vi "Test_URI_Class_SetPath.vi"(8 "error in (no error)":errorcluster) -> (0 "error out":errorcluster)   [LabVIEW 2013]
uses:
  source/uri/URI.lvclass/URI.ctl
  source/components/path/URI-Component.Path.lvclass/URI-Component.Path.ctl
  source/components/path/Get Segments.vi
  <vilib>/addons/_JKI Toolkits/Caraya/classes/Assert/Assert Equal Value_Variant.vi
  <vilib>/addons/_JKI Toolkits/Caraya/classes/Assert/Assert Error.vi
  source/components/path/Get base-path.vi
  source/components/path/Get path (absolute).vi
  source/components/path/Get path (relative-base).vi
  <vilib>/addons/_JKI Toolkits/Caraya/classes/Test/Test.lvclass
  <vilib>/addons/_JKI Toolkits/Caraya/classes/Assert/Assert.lvclass
  source/uri/URI.lvclass
panel:
  out "Segments":string[](array[string])
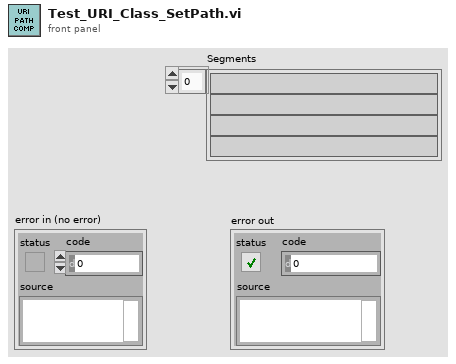
[diagram p1: front panel]
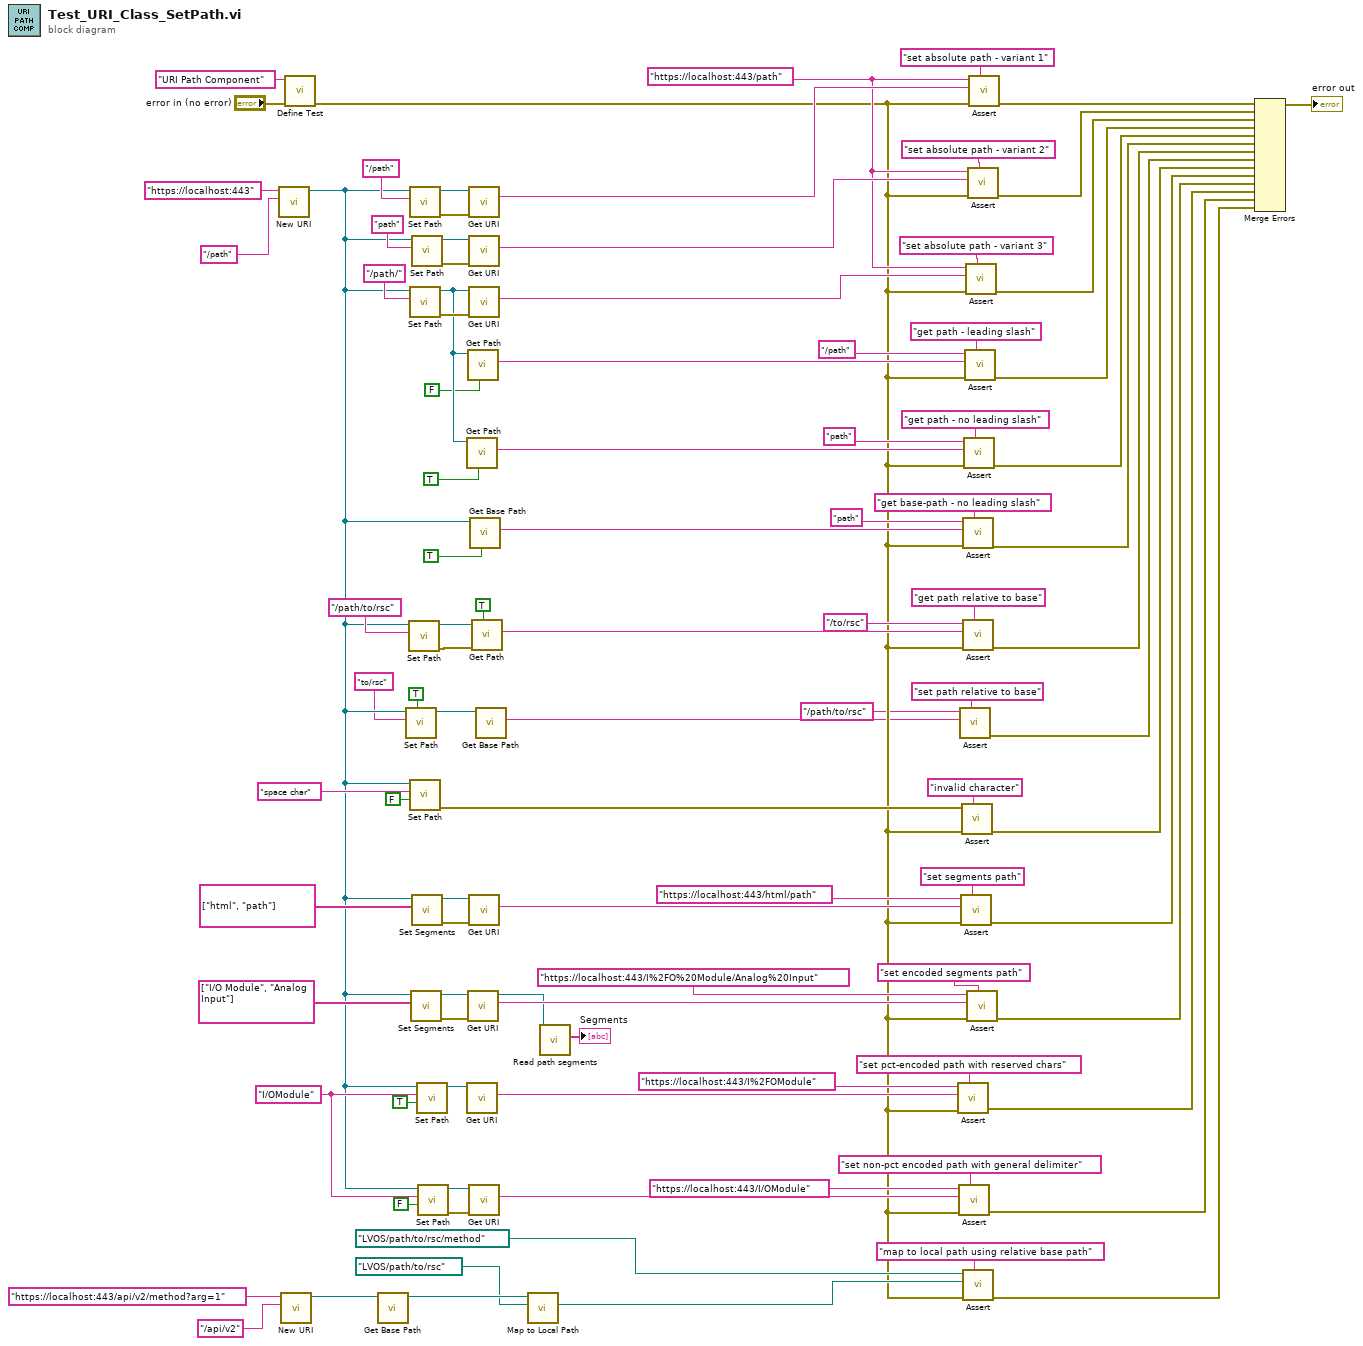
[diagram p0: block diagram]
diagram:
  w75 = "I/OModule" ("URI")
  w90 = "https://localhost:443/path" ("URI")
  n1 = call "New URI.vi"("base-path"="/path" ("URI"), "URI"="https://localhost:443") -> ("URI"=w6:refnum<class "URI.lvclass">)  [unwired: 8 in, 1 out]
  n2 = call "New URI.vi"("base-path"="/api/v2" ("URI"), "URI"="https://localhost:443/api/v2/method?arg=1") -> ("URI"=w22:refnum<class "URI.lvclass">)  [unwired: 8 in, 1 out]
  n3 = call <vilib>:"Define Test.vi"("error in (no error)"="error in (no error)", "Label (VI Title)"="URI Path Component") -> ("error out"=w11:errorcluster)  [unwired: 8 in, 1 out]
  n4 = call "Get Base Path.vi"("URI in"=w22) -> ("URI out"=w24:refnum<class "URI.lvclass">)  [unwired: 8 in, 2 out]
  n5 = call "Set Path.vi"("Use base-path?"=TRUE, "path"="to/rsc" ("URI"), "URI in"=w6) -> ("URI out"=w4:refnum<class "URI.lvclass">)  [unwired: 7 in, 1 out]
  n6 = call "Set Path.vi"("path"="/path/to/rsc" ("URI"), "URI in"=w6) -> ("error out"=w14:errorcluster, "URI out"=w16:refnum<class "URI.lvclass">)  [unwired: 8 in]
  n7 = call "Set Path.vi"("path"="/path" ("URI"), "URI in"=w6) -> ("error out"=w64:errorcluster, "URI out"=w63:refnum<class "URI.lvclass">)  [unwired: 8 in]
  n8 = call "Set Path.vi"("path"="/path/" ("URI"), "URI in"=w6) -> ("error out"=w59:errorcluster, "URI out"=w44:refnum<class "URI.lvclass">)  [unwired: 8 in]
  n9 = call "Set Path.vi"("Encode?"=FALSE, "path"="space char" ("URI"), "URI in"=w6) -> ("error out"=w73:errorcluster)  [unwired: 7 in, 1 out]
  n10 = call "Set Segments.vi"("Segments"=string[] ["I/O Module", "Analog Input"], "URI in"=w6) -> ("error out"=w54:errorcluster, "URI out"=w53:refnum<class "URI.lvclass">)  [unwired: 8 in]
  n11 = call "Set Path.vi"("path"="path" ("URI"), "URI in"=w6) -> ("error out"=w62:errorcluster, "URI out"=w61:refnum<class "URI.lvclass">)  [unwired: 8 in]
  n12 = call "Set Segments.vi"("Segments"=string[] ["html", "path"], "URI in"=w6) -> ("error out"=w55:errorcluster, "URI out"=w56:refnum<class "URI.lvclass">)  [unwired: 8 in]
  n13 = call "Set Path.vi"("Encode?"=TRUE, "path"=w75, "URI in"=w6) -> ("URI out"=w77:refnum<class "URI.lvclass">)  [unwired: 7 in, 1 out]
  n14 = call "Set Path.vi"("Encode?"=FALSE, "path"=w75, "URI in"=w6) -> ("error out"=w71:errorcluster, "URI out"=w70:refnum<class "URI.lvclass">)  [unwired: 7 in]
  n15 = call "Get Path.vi"("Strip lead \"/\" (F)"=TRUE ("Strip lead \"/\" (F)"), "URI in"=w44) -> ("path"=w35:string)  [unwired: 7 in, 2 out]
  n16 = call "Get URI.vi"("URI in"=w77) -> ("URI String"=w80:string)  [unwired: 8 in, 2 out]
  n17 = call "Get Path.vi"("Strip lead \"/\" (F)"=FALSE ("Strip lead \"/\" (F)"), "URI in"=w44) -> ("path"=w40:string)  [unwired: 7 in, 2 out]
  n18 = call "Get URI.vi"("error in (no error)"=w54, "URI in"=w53) -> ("URI String"=w47:string, "URI"=w46:refnum<class "URI.lvclass">)  [unwired: 7 in, 1 out]
  n19 = call "Get URI.vi"("error in (no error)"=w64, "URI in"=w63) -> ("URI String"=w94:string)  [unwired: 7 in, 2 out]
  n20 = call "Get URI.vi"("error in (no error)"=w62, "URI in"=w61) -> ("URI String"=w91:string)  [unwired: 7 in, 2 out]
  n21 = call "Get URI.vi"("error in (no error)"=w59, "URI in"=w44) -> ("URI String"=w89:string)  [unwired: 7 in, 2 out]
  n22 = call "Get URI.vi"("error in (no error)"=w55, "URI in"=w56) -> ("URI String"=w83:string)  [unwired: 7 in, 2 out]
  n23 = call "Get URI.vi"("error in (no error)"=w71, "URI in"=w70) -> ("URI String"=w66:string)  [unwired: 7 in, 2 out]
  n24 = call "Get Base Path.vi"("Strip lead \"/\" (F)"=TRUE ("Strip lead \"/\" (F)"), "URI in"=w6) -> ("base-path"=w28:string)  [unwired: 7 in, 2 out]
  n25 = call "Get Path.vi"("Use base-path?"=TRUE, "error in (no error)"=w14, "URI in"=w16) -> ("path"=w13:string)  [unwired: 6 in, 2 out]
  n26 = call "Get Base Path.vi"("URI in"=w4) -> ("base-path"=w3:string)  [unwired: 8 in, 2 out]
  n27 = call "Map to Local Path.vi"("Local Path"=path "LVOS/path/to/rsc", "URI in"=w24) -> ("Mapped Local Path"=w21:path)  [unwired: 6 in, 3 out]
  n28 = call "Read path segments.vi"("URI in"=w46) -> ("Segments"=→"Segments":string[])  [unwired: 8 in, 2 out]
  n29 = call-poly <vilib>:"Assert.vi"("Label"="set pct-encoded path with reserved chars" ("URI"), "error in (no error)"=w11, "Y"=w80, "X"="https://localhost:443/I%2FOModule" ("URI")) -> ("error out"=w49:errorcluster)  [unwired: 6 in, 1 out]
  n30 = call-poly <vilib>:"Assert.vi"("Label"="set non-pct encoded path with general delimiter" ("URI"), "error in (no error)"=w11, "Y"=w66, "X"="https://localhost:443/I/OModule" ("URI")) -> ("error out"=w67:errorcluster)  [unwired: 6 in, 1 out]
  n31 = call-poly <vilib>:"Assert.vi"("Label"="set path relative to base" ("URI"), "Y"=w3, "X"="/path/to/rsc" ("URI")) -> ("error out"=w7:errorcluster)  [unwired: 7 in, 1 out]
  n32 = call-poly <vilib>:"Assert.vi"("Label"="set segments path" ("URI"), "error in (no error)"=w11, "Y"=w83, "X"="https://localhost:443/html/path" ("URI")) -> ("error out"=w84:errorcluster)  [unwired: 6 in, 1 out]
  n33 = call-poly <vilib>:"Assert.vi"("Label"="invalid character" ("URI"), "error in (no error)"=w11, "Error?"=w73) -> ("error out"=w38:errorcluster)  [unwired: 7 in, 1 out]
  n34 = call-poly <vilib>:"Assert.vi"("Label"="get base-path - no leading slash" ("URI"), "error in (no error)"=w11, "Y"=w28, "X"="path" ("URI")) -> ("error out"=w25:errorcluster)  [unwired: 6 in, 1 out]
  n35 = call-poly <vilib>:"Assert.vi"("Label"="get path relative to base" ("URI"), "error in (no error)"=w11, "Y"=w13, "X"="/to/rsc" ("URI")) -> ("error out"=w10:errorcluster)  [unwired: 6 in, 1 out]
  n36 = call-poly <vilib>:"Assert.vi"("Label"="map to local path using relative base path" ("URI"), "error in (no error)"=w11, "Y"=w21, "X"=path "LVOS/path/to/rsc/method") -> ("error out"=w20:errorcluster)  [unwired: 6 in, 1 out]
  n37 = call-poly <vilib>:"Assert.vi"("Label"="get path - no leading slash" ("URI"), "error in (no error)"=w11, "Y"=w35, "X"="path" ("URI")) -> ("error out"=w33:errorcluster)  [unwired: 6 in, 1 out]
  n38 = call-poly <vilib>:"Assert.vi"("Label"="get path - leading slash" ("URI"), "error in (no error)"=w11, "Y"=w40, "X"="/path" ("URI")) -> ("error out"=w37:errorcluster)  [unwired: 6 in, 1 out]
  n39 = call-poly <vilib>:"Assert.vi"("Label"="set absolute path - variant 3" ("URI"), "error in (no error)"=w11, "Y"=w89, "X"=w90) -> ("error out"=w87:errorcluster)  [unwired: 6 in, 1 out]
  n40 = call-poly <vilib>:"Assert.vi"("Label"="set encoded segments path" ("URI"), "error in (no error)"=w11, "Y"=w47, "X"="https://localhost:443/I%2FO%20Module/Analog%20Input" ("URI")) -> ("error out"=w48:errorcluster)  [unwired: 6 in, 1 out]
  n41 = call-poly <vilib>:"Assert.vi"("Label"="set absolute path - variant 2" ("URI"), "error in (no error)"=w11, "Y"=w91, "X"=w90) -> ("error out"=w88:errorcluster)  [unwired: 6 in, 1 out]
  n42 = call-poly <vilib>:"Assert.vi"("Label"="set absolute path - variant 1" ("URI"), "error in (no error)"=w11, "Y"=w94, "X"=w90) -> ("error out"=w95:errorcluster)  [unwired: 6 in, 1 out]
  n43 = Merge Errors(w95, w88, w87, w37, w33, w25, w10, w7, w38, w84, w48, w49, w67, w20) -> (→"error out":errorcluster)
